vi "Simple LabVIEW Build.vi"() -> ()   [LabVIEW 2014]
uses:
  Controls/Cron String - STYP.ctl
  Controls/Source Code Control Selection - STYP.ctl
  Shared/Controls/LabVIEW Build - STYP.ctl
  Actors/LabVIEW Build/LabVIEW Build.lvclass
  Actors/CI Project/CI Project.lvclass
  Actors/Job Initialize/Job Initialize.lvclass
panel:
  in  "Source Code Poll":T1
  in  "Notification (Separate by Space)":string="brandyn.adderley@ni.com"
  in  "Artifact Days":i32=15
  in  "Project Name":string="LAF Test"
  in  "Hostname":string="10.211.55.18:8080"
  in  "Build Spec":string="Test LabVIEW Launcher"
  in  "Project Path":path=path "C:/Projects/LabVIEW Continuous Integration/LabVIEW Continuous Integration.lvproj"
  in  "Build Trigger":T2={"Day of Week"=enum."Everyday", "Hour"=23, "Enable?"=TRUE} {"Hour" min=0 max=23}
  out "Post Result":string
  out "error out":errorcluster
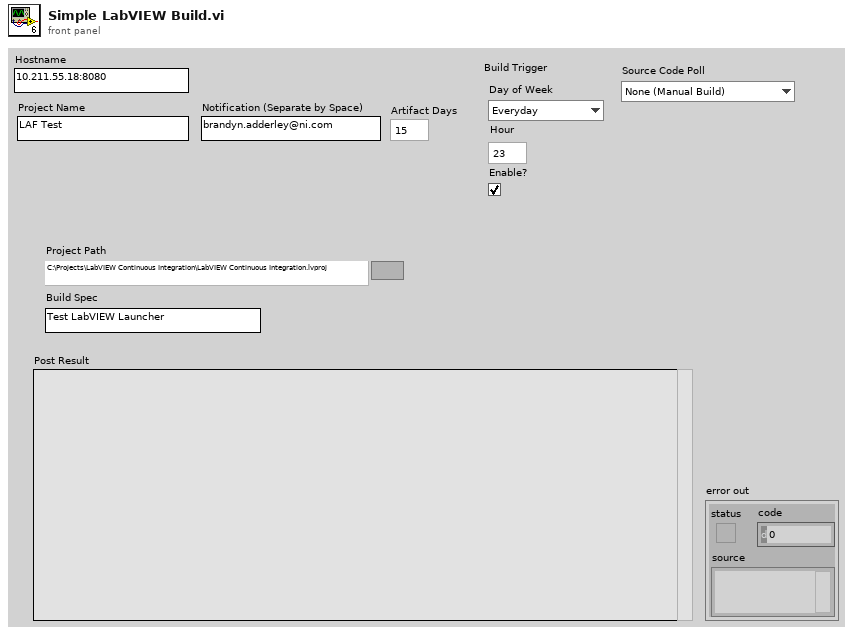
[diagram p1: front panel]
types:
  T1 = typedef "Source Code Control Selection - STYP.ctl" = enum16{"None (Manual Build)", "Every 15 Minutes", "Every 30 Minutes", "Every 45 Minutes", "Every Hour", "Every 2 Hours", "Everyday "}
  T2 = typedef "Cron String - STYP.ctl" = cluster{"Day of Week":enum16{"Everyday", "Sunday", "Monday", "Tuesday", "Wednesday", "Thursday", "Friday", "Saturday"}, "Hour":i32, "Enable?":bool}
  T3 = typedef "LabVIEW Build - STYP.ctl" = cluster{"Executor_Number":string, "Workspace_Path":string, "Build_Spec":string, "Project_Path":string, "Auto_Version_Increment":bool}
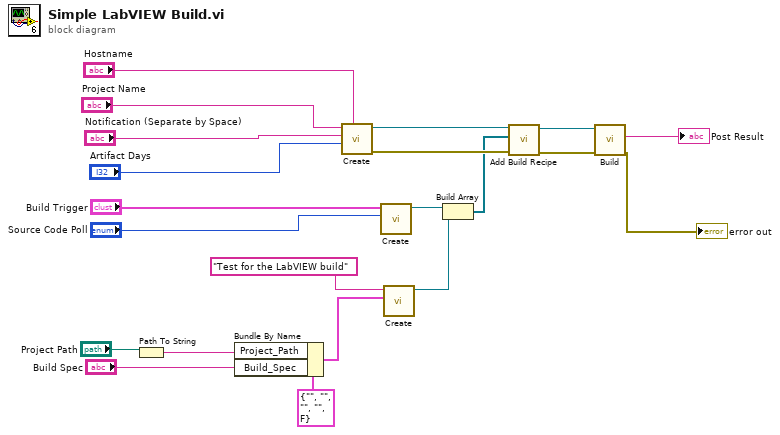
[diagram p0: block diagram]
diagram:
  n1 = Path To String(path="Project Path") -> (string=w4:string)
  n2 = Bundle By Name(cluster=T3 {"Executor_Number"="", "Workspace_Path"="", "Build_Spec"="", "Project_Path"="", "Auto_Version_Increment"=FALSE} ("LabVIEW Build"), "Project_Path"=w4, "Build_Spec"="Build Spec") -> (w1:T3)
  n3 = call "Create.vi"("HostName"="Hostname", "Artifact Days"="Artifact Days", "Notification"="Notification (Separate by Space)", "Project Name"="Project Name") -> ("error out"=w20:errorcluster, "CI Project out"=w21:refnum<class "CI Project.lvclass">)  [unwired: 6 in]
  n4 = call "Create.vi"("Source Code Poll"="Source Code Poll", "Build Trigger"="Build Trigger") -> ("Job Initialize out"=w11:refnum<class "Job Initialize.lvclass">)  [unwired: 8 in, 1 out]
  n5 = call "Create.vi"("LabVIEW Build"=w1, "Description"="Test for the LabVIEW build") -> ("LabVIEW Build out"=w19:refnum<class "LabVIEW Build.lvclass">)  [unwired: 8 in, 1 out]
  n6 = Build Array(w11, w19) -> (w18:refnum<class "Build Job.lvclass">[])
  n7 = call "Add Build Recipe.vi"("error in (no error)"=w20, "Build Recipe"=w18, "CI Project in"=w21) -> ("error out"=w16:errorcluster, "CI Project out"=w17:refnum<class "CI Project.lvclass">)  [unwired: 7 in]
  n8 = call "Build.vi"("error in (no error)"=w16, "CI Project in"=w17) -> ("error out"=→"error out":errorcluster, "Log Text"=→"Post Result":string)  [unwired: 7 in, 1 out]
